vi "test-QDSL.vi"() -> ()   [LabVIEW 2011]
panel:
  in  "Indium Flow 2":dbl=37.6
  in  "Ga Flow 3":dbl=4.2
  in  "Ga Flow 2":dbl=4.2
  in  "Ga Flow 1":dbl=4.2
  in  "Indium Flow":dbl=37.6
  in  "Number of \nGrowth Steps":i32=10
  out "step number":i32
  in  "As_Gas Flow":dbl=3.5
  in  "Manifold H2 Flow":dbl=720.0
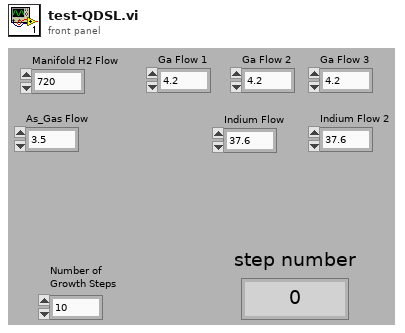
[diagram p1: front panel]
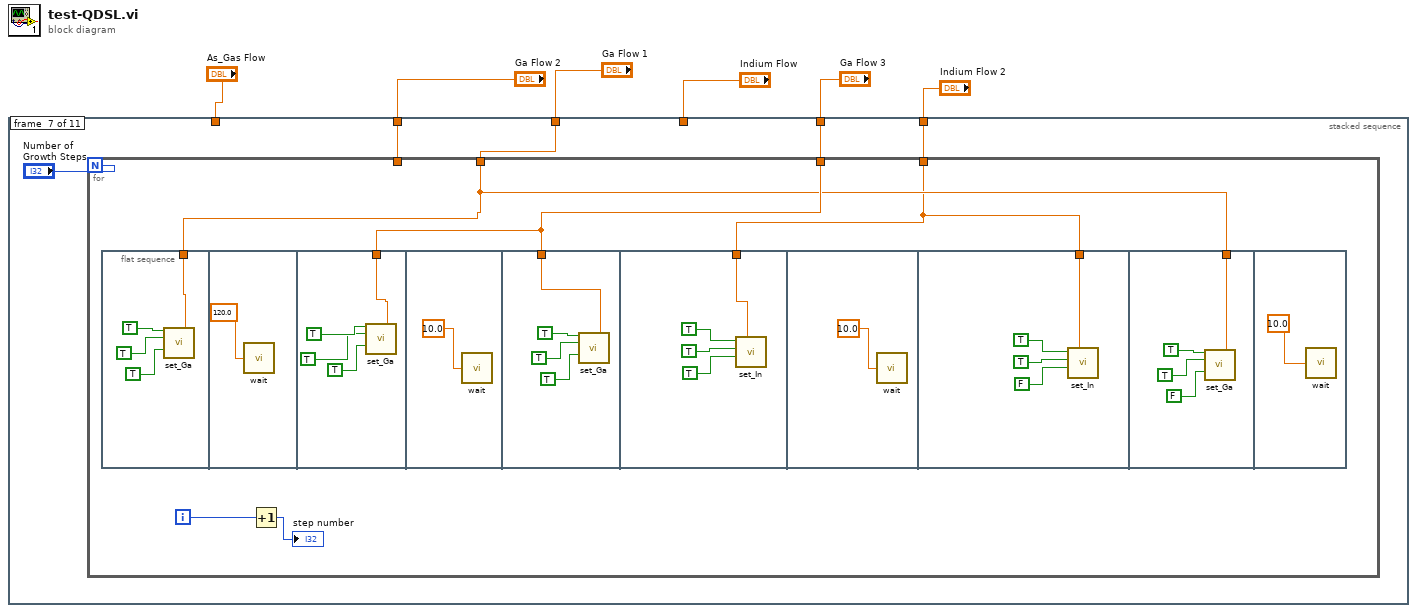
[diagram p0: block diagram]
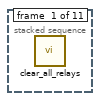
[diagram p2: hidden frame]
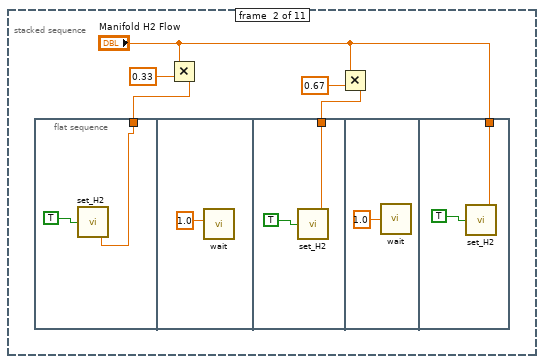
[diagram p3: hidden frame]
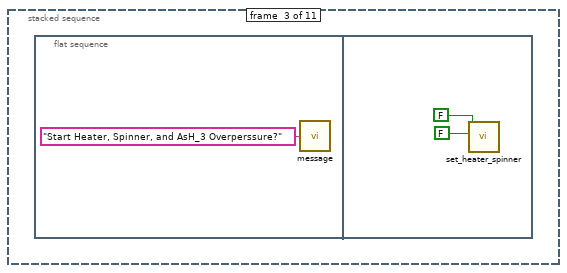
[diagram p4: hidden frame]
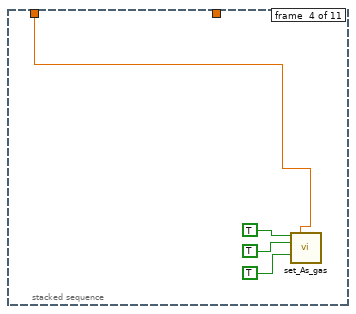
[diagram p5: hidden frame]
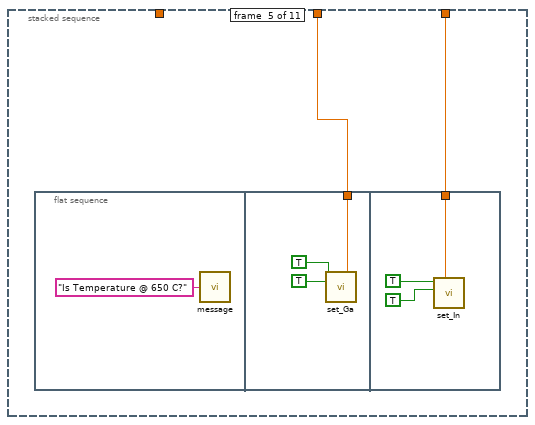
[diagram p6: hidden frame]
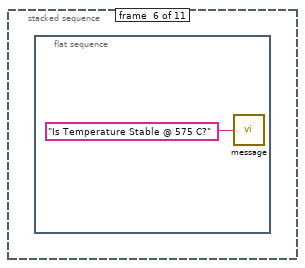
[diagram p7: hidden frame]
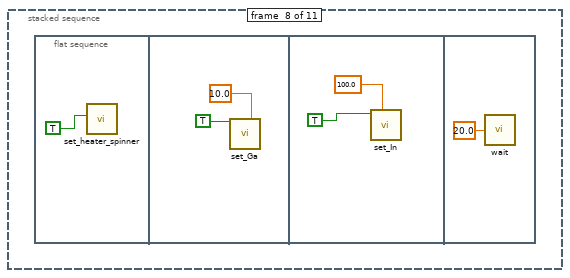
[diagram p8: hidden frame]
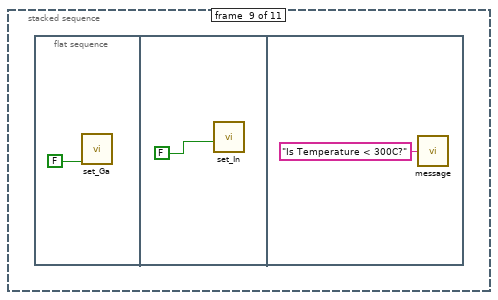
[diagram p9: hidden frame]
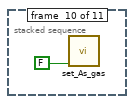
[diagram p10: hidden frame]
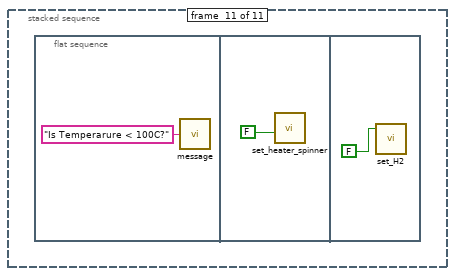
[diagram p11: hidden frame]
diagram:
  n1 = stacked-sequence {
    tunnel: "Ga Flow 1" -> [_ _ _ _ w28 _ w40 _ _ _ _]
    tunnel: "As_Gas Flow" -> [_ _ _ w23 _ _ _ _ _ _ _]
    tunnel: "Indium Flow" -> [_ _ _ _ w27 _ _ _ _ _ _]
    tunnel: "Ga Flow 2" -> [_ _ _ _ _ _ w39 _ _ _ _]
    tunnel: "Ga Flow 3" -> [_ _ _ _ _ _ w38 _ _ _ _]
    tunnel: "Indium Flow 2" -> [_ _ _ _ _ _ w37 _ _ _ _]
    frame #0 {
      n2 = call "clear_all_relays.vi"() -> ()  [unwired: 2 out]
    }
    frame #1 {
      n3 = flat-sequence {
        tunnel: w11 -> [w12]
        tunnel: w9 -> [w15]
        tunnel: "Manifold H2 Flow" -> [w18]
        frame #0 {
          n4 = call "set_H2.vi"("Manifold H2 Flow"=w12, "H2 Active"=TRUE) -> ()  [unwired: 2 in, 2 out]
        }
        frame #1 {
          n5 = call "wait.vi"("Wait (s)"=1.0) -> ()
        }
        frame #2 {
          n6 = call "set_H2.vi"("Manifold H2 Flow"=w15, "H2 Active"=TRUE) -> ()  [unwired: 2 in, 2 out]
        }
        frame #3 {
          n7 = call "wait.vi"("Wait (s)"=1.0) -> ()
        }
        frame #4 {
          n8 = call "set_H2.vi"("Manifold H2 Flow"=w18, "H2 Active"=TRUE) -> ()  [unwired: 2 in, 2 out]
        }
      }
      n9 = Multiply(x="Manifold H2 Flow", y=0.33) -> (x*y=w11:dbl)
      n10 = Multiply(x="Manifold H2 Flow", y=0.67) -> (x*y=w9:dbl)
    }
    frame #2 {
      n11 = flat-sequence {
        frame #0 {
          n12 = call "message.vi"("message"="Start Heater, Spinner, and AsH_3 Overperssure?") -> ()
        }
        frame #1 {
          n13 = call "set_heater_spinner.vi"("Spinner"=FALSE, "Heater"=FALSE) -> ()  [unwired: 1 in, 7 out]
        }
      }
    }
    frame #3 {
      n14 = call "set_As_gas.vi"("As_Gas Active"=TRUE, "As_Gas Flow"=w23, "As_Gas In"=TRUE, "As_Gas Run"=TRUE) -> ()  [unwired: 2 in, 10 out]
    }
    frame #4 {
      n15 = flat-sequence {
        tunnel: w28 -> [w30]
        tunnel: w27 -> [w33]
        frame #0 {
          n16 = call "message.vi"("message"="Is Temperature @ 650 C?") -> ()
        }
        frame #1 {
          n17 = call "set_Ga.vi"("Ga Active"=TRUE, "Ga Flow 1"=w30, "Ga Bubbler"=TRUE) -> ()  [unwired: 5 in, 8 out]
        }
        frame #2 {
          n18 = call "set_In.vi"("Indium Flow"=w33, "In Bubbler"=TRUE ("Ga Bubbler"), "In Active"=TRUE ("Ga Active")) -> ()  [unwired: 2 in, 5 out]
        }
      }
    }
    frame #5 {
      n19 = flat-sequence {
        frame #0 {
          n20 = call "message.vi"("message"="Is Temperature Stable @ 575 C?") -> ()
        }
      }
    }
    frame #6 {
      n21 = for {
        N: "Number of \nGrowth Steps" -> [_]
        tunnel: w40 -> [w43]
        tunnel: w39 -> [_]
        tunnel: w38 -> [w44]
        tunnel: w37 -> [w42]
        i -> [w45]
        n22 = flat-sequence {
          tunnel: w43 -> [w47]
          tunnel: w44 -> [w52]
          tunnel: w44 -> [w57]
          tunnel: w42 -> [w61]
          tunnel: w42 -> [w66]
          tunnel: w43 -> [w70]
          frame #0 {
            n23 = call "set_Ga.vi"("Ga Active"=TRUE ("P_Gas Active"), "Ga Flow 1"=w47, "Ga Bubbler"=TRUE ("P_Gas In"), "Ga Run"=TRUE ("P_Gas Run")) -> ()  [unwired: 4 in, 8 out]
          }
          frame #1 {
            n24 = call "wait.vi"("Wait (s)"=120.0) -> ()
          }
          frame #2 {
            n25 = call "set_Ga.vi"("Ga Active"=TRUE ("P_Gas Active"), "Ga Flow 1"=w52, "Ga Bubbler"=TRUE ("P_Gas In"), "Ga Run"=TRUE ("P_Gas Run")) -> ()  [unwired: 4 in, 8 out]
          }
          frame #3 {
            n26 = call "wait.vi"("Wait (s)"=10.0) -> ()
          }
          frame #4 {
            n27 = call "set_Ga.vi"("Ga Active"=TRUE ("P_Gas Active"), "Ga Flow 1"=w57, "Ga Bubbler"=TRUE ("P_Gas In"), "Ga Run"=TRUE ("P_Gas Run")) -> ()  [unwired: 4 in, 8 out]
          }
          frame #5 {
            n28 = call "set_In.vi"("Indium Flow"=w61, "In Run"=TRUE ("P_Gas Run"), "In Bubbler"=TRUE ("P_Gas In"), "In Active"=TRUE ("P_Gas Active")) -> ()  [unwired: 1 in, 5 out]
          }
          frame #6 {
            n29 = call "wait.vi"("Wait (s)"=10.0) -> ()
          }
          frame #7 {
            n30 = call "set_In.vi"("Indium Flow"=w66, "In Run"=FALSE ("P_Gas Run"), "In Bubbler"=TRUE ("P_Gas In"), "In Active"=TRUE ("P_Gas Active")) -> ()  [unwired: 1 in, 5 out]
          }
          frame #8 {
            n31 = call "set_Ga.vi"("Ga Active"=TRUE ("P_Gas Active"), "Ga Flow 1"=w70, "Ga Bubbler"=TRUE ("P_Gas In"), "Ga Run"=FALSE ("P_Gas Run")) -> ()  [unwired: 4 in, 8 out]
          }
          frame #9 {
            n32 = call "wait.vi"("Wait (s)"=10.0) -> ()
          }
        }
        n33 = Increment(x=w45) -> (x+1=→"step number":i32)
      }
    }
    frame #7 {
      n34 = flat-sequence {
        frame #0 {
          n35 = call "set_heater_spinner.vi"("Spinner"=TRUE ("Ga Active")) -> ()  [unwired: 2 in, 7 out]
        }
        frame #1 {
          n36 = call "set_Ga.vi"("Ga Active"=TRUE, "Ga Flow 1"=10.0) -> ()  [unwired: 6 in, 8 out]
        }
        frame #2 {
          n37 = call "set_In.vi"("Indium Flow"=100.0 ("Aluminum Flow"), "In Active"=TRUE ("Ga Active")) -> ()  [unwired: 3 in, 5 out]
        }
        frame #3 {
          n38 = call "wait.vi"("Wait (s)"=20.0) -> ()
        }
      }
    }
    frame #8 {
      n39 = flat-sequence {
        frame #0 {
          n40 = call "set_Ga.vi"("Ga Remote"=FALSE) -> ()  [unwired: 7 in, 8 out]
        }
        frame #1 {
          n41 = call "set_In.vi"("In Run"=FALSE ("Ga Remote")) -> ()  [unwired: 4 in, 5 out]
        }
        frame #2 {
          n42 = call "message.vi"("message"="Is Temperature < 300C?") -> ()
        }
      }
    }
    frame #9 {
      n43 = call "set_As_gas.vi"("As_Gas Remote"=FALSE) -> ()  [unwired: 5 in, 10 out]
    }
    frame #10 {
      n44 = flat-sequence {
        frame #0 {
          n45 = call "message.vi"("message"="Is Temperarure < 100C?") -> ()
        }
        frame #1 {
          n46 = call "set_heater_spinner.vi"("Heater/Spinner Remote"=FALSE) -> ()  [unwired: 2 in, 7 out]
        }
        frame #2 {
          n47 = call "set_H2.vi"("H2N2 Remote"=FALSE) -> ()  [unwired: 3 in, 2 out]
        }
      }
    }
  }
